vi "quad_max.vi"(1 "d":dbl, 2 "c":dbl, 3 "b":dbl, 4 "a":dbl) -> (0 "max":dbl)   [LabVIEW 2020]
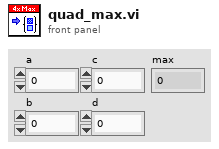
[diagram p1: front panel]
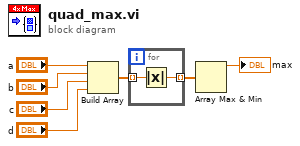
[diagram p0: block diagram]
diagram:
  n1 = Build Array("a", "b", "c", "d") -> (w7:dbl[])
  n2 = for {
    tunnel: w7 -> [w8] mode=indexing
    tunnel: [w9] -> w6 mode=indexing
    n3 = Absolute Value(x=w8) -> (abs(x)=w9:dbl)
  }
  n4 = Array Max & Min(array=w6) -> (max value=→"max":dbl)  [unwired: 3 out]
